vi "PH_BeamlineController.PC Set-PA DP Target.vi"(0 "i ref in":refnum<vi>, 2 "PA DP Targets":T1, 3 "Value":bool, 5 "error in (no error)":errorcluster) -> (14 "i ref out":refnum<vi>, 17 "PA DP Targets changed?":bool, 19 "error out":errorcluster)   [LabVIEW 2014, in "PH_BeamlineController.lvlib"]
doc: "This VI writes incoming Information to own Attributes if the new value differs from the stored."
uses:
  PH_BeamlineController.lvlib
  PH_BeamlineController.PA DP Targets.ctl
  PH_SystemInformation/PH_SystemInformationEnabling State.ctl
  PH_Beamline_Chief/PH_Beamline_Chief.Section.ctl
  PH_SystemInformation/PH_SystemInformation.lvlib
  PH_BeamlineInformation/PH_BeamlineInformation.lvlib
  PH_Beamline_Chief/PH_Beamline_Chief.lvlib
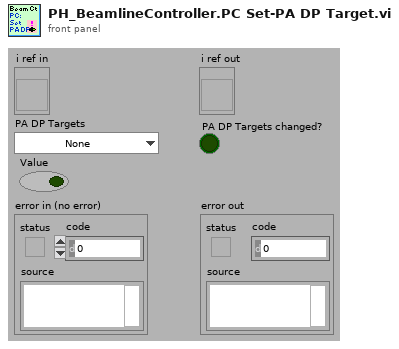
[diagram p1: front panel]
types:
  T1 = typedef "PH_BeamlineController.lvlib/PH_BeamlineController.PA DP Targets.ctl" = enum16{"None", "Dump PA Delayed Beam", "Dump PA Undelayed Beam", "Dumps PA Delayed and Undelayed Beam"}
  T2 = typedef "PH_Beamline_Chief.lvlib/PH_Beamline_Chief.Section.ctl" = enum16{"None", "YLF", "fs", "fs-YLF", "ns", "PA-Input", "PA-Undelay", "PA-Delay", "PA-before-Bypass", "PA", "PA-Bypass", "PA-Exit", "PA-LL", "LL", "PA-MA", "MA-Exit", "MA-Z6", "Z6", "MA-LB", "LB-TB2", "LB-TB3"}
  T3 = typedef "PH_SystemInformation.lvlib/PH_SystemInformationEnabling State.ctl" = i32
  T4 = enum16{"Laser", "PreAmp", "MainAmp", "Exp 1", "Exp 2", "Exp 3", "Exp 4"}
  T5 = typedef "PH_BeamlineController.lvlib/PH_BeamlineController.Sources.ctl" = enum16{"None", "YLF", "fs-Frontend", "ns-Frontend", "YLF and ns-Frontend", "fs- and ns-Frontend"}
  T6 = typedef "PH_BeamlineController.lvlib/PH_BeamlineController.Targets.ctl" = enum16{"None", "PreAmp", "Dump Exp Laserlab", "Exp Laserlab", "Calorimeter", "Dump Exp Laserbay", "Exp Laserbay", "Dump Exp Z6", "Exp Z6"}
  T7 = cluster{"Source":T5, "PA DP Target":T1, "Target":T6}
  T8 = typedef "PH_BeamlineController.lvlib/PH_BeamlineController.PA DP Target Attributes.ctl" = cluster{"Name":T1, "GUI Ref":refnum<vi>, "Current State":bool, "Wanted State":bool, "Enabled":bool}
  T9 = typedef "PH_BeamlineController.lvlib/PH_BeamlineController.i attribute.ctl" = cluster{"Vacuum Exp LB":cluster{"Channel":string, "Limit [mbar]":dbl, "Pressure [mbar]":dbl, "GUI Ref":refnum<vi>}, "Sources":T10[], "PA DP Targets":T8[], "Path":cluster{"Source":T5, "PA DP Target":T1, "Target":T6}, "Targets":cluster{"Name":T6, "GUI Ref":refnum<vi>, "Current State":bool, "Wanted State":bool, "Enabled":bool}[], "Status Tags":cluster{"Name":string, "Status":T11}[], "special GUI Refs":T12}
  T10 = typedef "PH_BeamlineController.lvlib/PH_BeamlineController.Source Attributes.ctl" = cluster{"Name":T5, "GUI Ref":refnum<vi>, "Current State":bool, "Wanted State":bool}
  T11 = typedef "PH_StatusHandler.lvlib/PH_StatusHandler.Status.ctl" = i16
  T12 = typedef "PH_BeamlineController.lvlib/PH_BeamlineController.special GUI Refs.ctl" = cluster{"PA-Backreflection-Meas":refnum<vi>, "fs_Synchrolock_Watch":refnum<vi>}
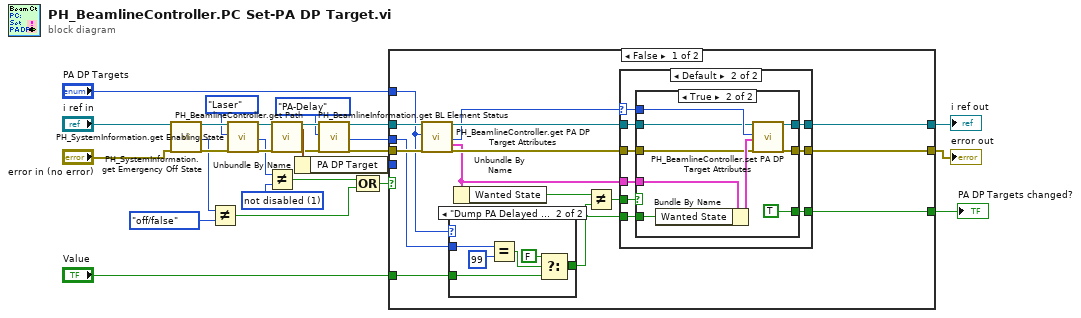
[diagram p0: block diagram]
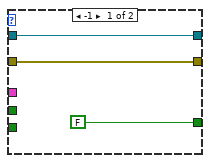
[diagram p3: hidden frame]
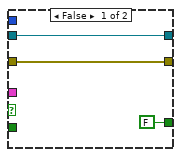
[diagram p4: hidden frame]
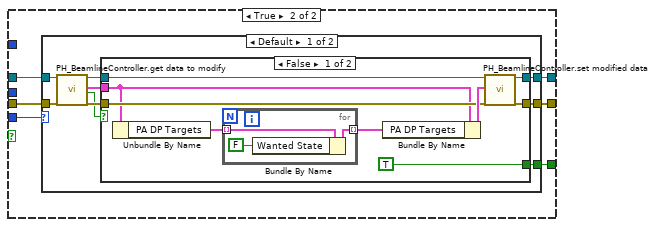
[diagram p5: hidden frame]
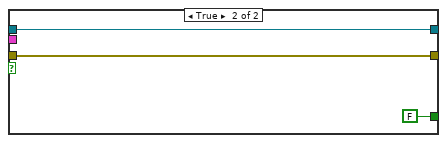
[diagram p6: hidden frame]
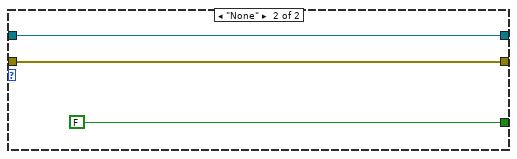
[diagram p7: hidden frame]
diagram:
  w14 = T3 1 items=["no info", "not disabled", "disabled"] ("y")
  n1 = call "PH_SystemInformation.get Emergency Off State.vi"("i ref in"="i ref in", "error in (no error)"="error in (no error)") -> ("i ref out"=w23:refnum<vi>, "Emergency Off State"=w13:enum16{"no info", "off/false", "Alarm"}, "error out"=w22:errorcluster)  [unwired: 15 in]
  n2 = Not Equal?(x=w13, y=enum16{"no info", "off/false", "Alarm"}."off/false") -> (x != y?=w10:bool)
  n3 = call "PH_SystemInformation.get Enabling State.vi"("i ref in"=w23, "Wanted State"=T4."Laser", "error in (no error)"=w22) -> ("i ref out"=w17:refnum<vi>, "Enabling State"=w12:T3, "error out"=w16:errorcluster)  [unwired: 14 in]
  n4 = Not Equal?(x=w12, y=w14) -> (x != y?=w11:bool)
  n5 = call "PH_BeamlineController.get Path.vi"("VI in"=w17, "error in (no error)"=w16) -> ("VI out"=w4:refnum<vi>, "Path"=w7:T7, "error out"=w6:errorcluster)  [unwired: 12 in, 3 out]
  n6 = Unbundle By Name(w7) -> ("PA DP Target"=w8:T1)
  n7 = call "PH_BeamlineInformation.get BL Element Status.vi"("VI in"=w4, "Beamline Element"=PH_Beamline_Chief.Section."PA-Delay", "error in (no error)"=w6) -> ("VI out"=w3:refnum<vi>, "Status"=w1:i32, "error out"=w5:errorcluster)  [unwired: 14 in]
  n8 = Compound Arithmetic op=OR(w11, w10) -> (w9:bool)
  n9 = case shown="False" w9 {
    tunnel: [w42 w75] -> w27
    tunnel: [w41 w76] -> w26
    tunnel: "PA DP Targets" -> [w31 _]
    tunnel: [w40 w74] -> w24
    tunnel: "Value" -> [w30 _]
    tunnel: w3 -> [w33 w77]
    tunnel: w5 -> [w32 w78]
    tunnel: w8 -> [_ w79]
    tunnel: w1 -> [w28 _]
    frame False {
      n10 = call "PH_BeamlineController.get PA DP Target Attributes.vi"("VI in"=w33, "PA DP Target"=w31, "error in (no error)"=w32) -> ("VI out"=w38:refnum<vi>, "PA DP Target Index"=w34:i32, "PA DP Target Attributes"=w37:T8, "error out"=w39:errorcluster)  [unwired: 13 in]
      n11 = case shown="\"Dump PA Delayed Beam\", \"Dump PA Undelayed Beam\"" w31 {
        tunnel: w28 -> [_ w49]
        tunnel: w30 -> [w43 w46]
        tunnel: [w43 w45] -> w29
        frame Default {
        }
        frame "Dump PA Delayed Beam", "Dump PA Undelayed Beam" {
          n12 = Equal?(x=w49, y=99) -> (x = y?=w47:bool)
          n13 = Select(t=FALSE, s=w47, f=w46) -> (s? t:f=w45:bool)
        }
      }
      n14 = Unbundle By Name(w37) -> ("Wanted State"=w36:bool)
      n15 = Not Equal?(x=w36, y=w29) -> (x != y?=w35:bool)
      n16 = case shown="Default" w34 {
        selector: w34 -> [_ w53]
        tunnel: [w51 w61] -> w42
        tunnel: [w52 w60] -> w41
        tunnel: w39 -> [w51 w59]
        tunnel: w38 -> [w52 w58]
        tunnel: w29 -> [_ w57]
        tunnel: w37 -> [_ w56]
        tunnel: w35 -> [_ w55]
        tunnel: [FALSE w54] -> w40
        frame -1 {
        }
        frame Default {
          n17 = case shown="True" w55 {
            tunnel: [w64 w68] -> w60
            tunnel: [w63 w67] -> w61
            tunnel: w59 -> [w63 w65]
            tunnel: w58 -> [w64 w66]
            tunnel: w53 -> [_ w73]
            tunnel: w56 -> [_ w72]
            tunnel: w57 -> [_ w70]
            tunnel: [FALSE TRUE] -> w54
            frame False {
            }
            frame True {
              n18 = Bundle By Name(cluster=w72, "Wanted State"=w70) -> (w71:T8)
              n19 = call "PH_BeamlineController.set PA DP Target Attributes.vi"("VI in"=w66, "PA DP Target Index"=w73, "Changed PA DP Target Attributes"=w71, "error in (no error)"=w65) -> ("VI out"=w68:refnum<vi>, "error out"=w67:errorcluster)  [unwired: 14 in]
            }
          }
        }
      }
    }
    frame True {
      n20 = case shown="Default" w79 {
        tunnel: w78 -> [w83 w105]
        tunnel: w77 -> [w84 w106]
        tunnel: [w82 w106] -> w76
        tunnel: [w81 w105] -> w75
        tunnel: [w80 FALSE] -> w74
        frame Default {
          n21 = call "PH_BeamlineController.get data to modify.vi"("i ref in"=w84, "error in (no error)"=w83) -> ("i ref out"=w88:refnum<vi>, "i attribute"=w86:T9, "timed out"=w85:bool, "error out"=w87:errorcluster)  [unwired: 14 in]
          n22 = case shown="False" w85 {
            tunnel: w88 -> [w94 w103]
            tunnel: [w97 w103] -> w82
            tunnel: w87 -> [w93 w102]
            tunnel: [w96 w102] -> w81
            tunnel: w86 -> [w92 _]
            tunnel: [TRUE FALSE] -> w80
            frame False {
              n23 = Unbundle By Name(w92) -> ("PA DP Targets"=w91:T8[])
              n24 = for {
                tunnel: w91 -> [w100] mode=indexing
                tunnel: [w99] -> w90 mode=indexing
                n25 = Bundle By Name(cluster=w100, "Wanted State"=FALSE) -> (w99:T8)
              }
              n26 = Bundle By Name(cluster=w92, "PA DP Targets"=w90) -> (w95:T9)
              n27 = call "PH_BeamlineController.set modified data.vi"("i ref in"=w94, "i attribute"=w95, "error in (no error)"=w93) -> ("i ref out"=w97:refnum<vi>, "error out"=w96:errorcluster)  [unwired: 15 in]
            }
            frame True {
            }
          }
        }
        frame "None" {
        }
      }
    }
  }
  "error out" <- w27
  "i ref out" <- w26
  "PA DP Targets changed?" <- w24
